vi "CreateEventTestListener.vi"(8 "error in (no error)":errorcluster) -> (0 "error out":errorcluster, 3 "EventTestListener":refnum<class "EventTestListener.lvclass">)   [LabVIEW 2019, in "TestExplorer.lvlib" / "EventTestListener.lvclass"]
uses:
  EventTestListener.lvclass
  FailureEventData.ctl
  TestCase/TestCase/TestCase.lvclass
  TestEndedEventData.ctl
  EventTestListener.lvclass/EventTestListener.ctl
  TestCase/Fact/Fact.lvclass
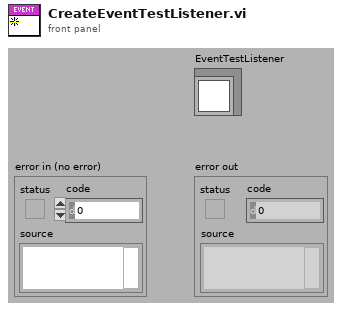
[diagram p1: front panel]
types:
  T1 = typedef "TestExplorer.lvlib/EventTestListener.lvclass/TestEndedEventData.ctl" = cluster{"TestCase":refnum<class "TestCase.lvclass">, "Time":dbl}
  T2 = typedef "TestExplorer.lvlib/EventTestListener.lvclass/FailureEventData.ctl" = cluster{"TestCase":refnum<class "TestCase.lvclass">, "Failure":errorcluster, "Time":dbl}
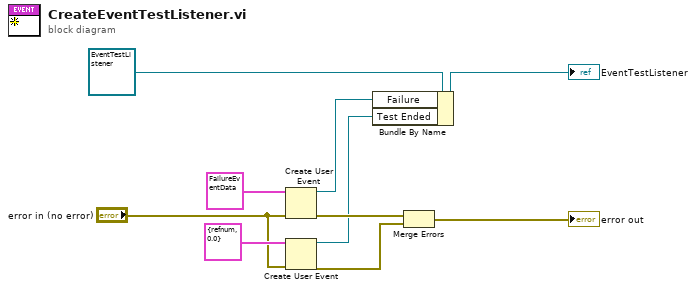
[diagram p0: block diagram]
diagram:
  n1 = Create User Event(user event datatype=T2 {"TestCase"=refnum, "Failure"={"status"=TRUE, "code"=-8000, "source"="TestResultTest.lvlib:testPassed.vi<ERR>\nFailed asserting that actual size 0 matches expected size 1."}, "Time"=0.08753380000052857} ("FailureEventData"), error in="error in (no error)") -> (user event=w7:refnum<user-event>, error out=w4:errorcluster)
  n2 = Create User Event(user event datatype=T1 {"TestCase"=refnum, "Time"=0.0} ("FailureEventData"), error in="error in (no error)") -> (user event=w1:refnum<user-event>, error out=w3:errorcluster)
  n3 = Bundle By Name(cluster=refnum<class "EventTestListener.lvclass"> refnum ("EventTestListener In"), "Failure"=w7, "Test Ended"=w1) -> (→"EventTestListener":refnum<class "EventTestListener.lvclass">)
  n4 = Merge Errors(w4, w3) -> (→"error out":errorcluster)
